vi "copy HPLC data.vi"(4 "Backup location":path, 6 "Backup?":bool, 8 "error in":errorcluster, 9 "Experiment name":string, 10 "Experiment folder":path, 11 "HPLC folder":path=path "\\\\ECHEMHPLC-PC\\Chem32/1/DATA/DEFAULT.D") -> (0 "error out":errorcluster)   [LabVIEW 2017]
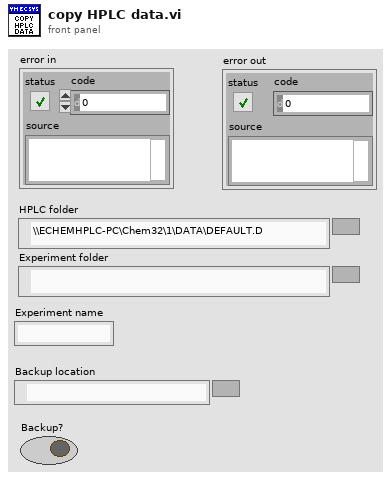
[diagram p1: front panel]
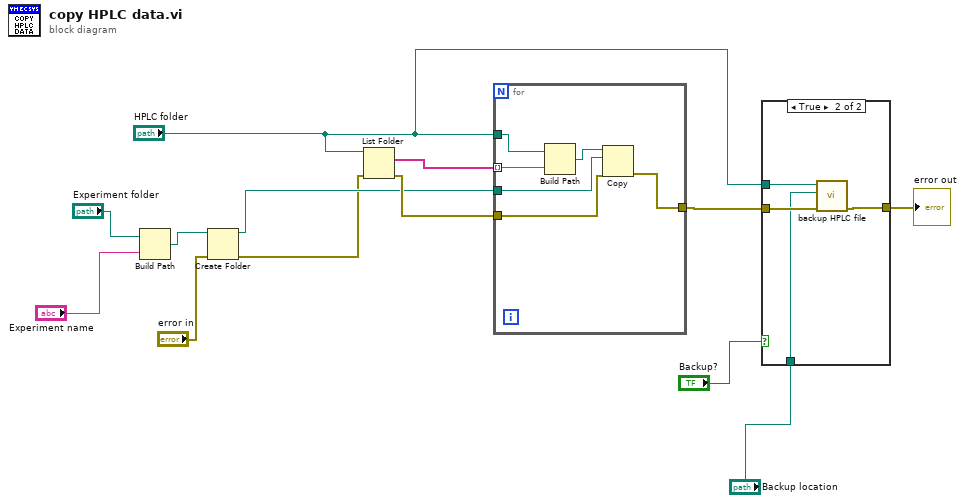
[diagram p0: block diagram]
diagram:
  n1 = Build Path(base path="Experiment folder", name or relative path="Experiment name") -> (appended path=w10:path)
  n2 = Create Folder(path (use dialog)=w10, error in="error in") -> (created path=w9:path, error out=w8:errorcluster)  [unwired: 1 in, 1 out]
  n3 = List Folder(path="HPLC folder", error in=w8) -> (filenames=w13:string[], error out=w12:errorcluster)  [unwired: 2 in, 2 out]
  n4 = for {
    tunnel: "HPLC folder" -> [w19]
    tunnel: w13 -> [w18] mode=indexing
    tunnel: w9 -> [w16]
    tunnel: w12 -> [w15]
    tunnel: [w14] -> w5
    n5 = Build Path(base path=w19, name or relative path=w18) -> (appended path=w17:path)
    n6 = Copy(8:w15, 10:w16, 11:w17) -> (0:w14:errorcluster)  [unwired: 2 in, 2 out]
  }
  n7 = case shown="True" "Backup?" {
    tunnel: w5 -> [w20 w24]
    tunnel: [w20 w23] -> w4
    tunnel: "HPLC folder" -> [_ w22]
    tunnel: "Backup location" -> [_ w21]
    frame False {
    }
    frame True {
      n8 = call "backup HPLC file.vi"("error in (no error)"=w24, "Backup location"=w21, "HPLC"=w22) -> ("error out"=w23:errorcluster)  [unwired: 8 in]
    }
  }
  "error out" <- w4
